vi "ArmLiftConstants.vi"() -> (0 "Starting Angle":dbl=-79.0, 2 "LiftConversionFactor":dbl=0.7322802197, 3 "StartingArmPos":dbl, 4 "Default Angle":dbl=-79.0)   [LabVIEW 2020]
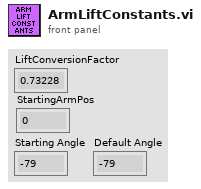
[diagram p1: front panel]
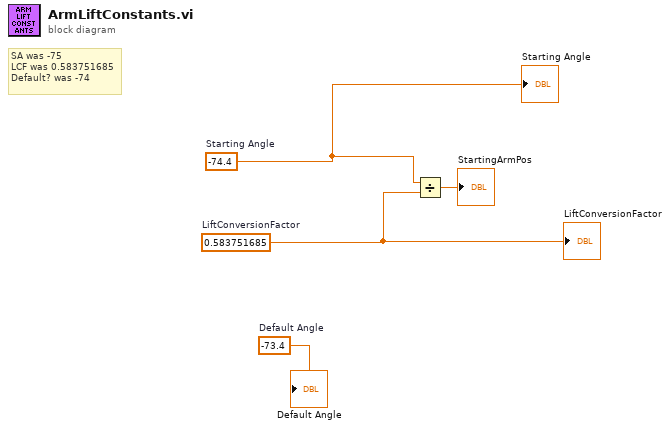
[diagram p0: block diagram]
diagram:
  w1 = -73.4  # Default Angle
  w4 = -74.4  # Starting Angle
  w3 = 0.583751685  # LiftConversionFactor
  # "SA was -75\nLCF was 0.583751685\nDefault? was -74"
  n1 = Divide(x=w4, y=w3) -> (x/y=→"StartingArmPos":dbl)
  "LiftConversionFactor" <- w3
  "Starting Angle" <- w4
  "Default Angle" <- w1
